vi "Signal-Generator.vi"() -> ()   [LabVIEW 2020]
uses:
  <vilib>/Analysis/1siggen.llb/Ramp Pattern by Samples.vi
  <vilib>/Analysis/2dsp.llb/Real FFT.vi
  <vilib>/Analysis/1siggen.llb/General Gauss-Mod Sine.vi
  <vilib>/Analysis/1siggen.llb/General Gaussian Monopulse.vi
  <vilib>/Analysis/1siggen.llb/General Aperiodic Triangle.vi
  <vilib>/Analysis/1siggen.llb/General Periodic Sinc.vi
  <vilib>/Analysis/NI_AALBase.lvlib
  <vilib>/Analysis/NI_AALPro.lvlib
panel:
  out "FFT":dbl[](graph)
  in  "dt":dbl=0.1
  in  "Delay":i32=50
  in  "SigFrequency":dbl=1.0 format="%.2f"
  in  "Samples":i32=256
  in  "Duration":dbl=1.0 format="%0.2f"
  in  "dc offset":dbl format="%0.2f"
  in  "Phase":dbl format="%0.2f"
  in  "Amplitude":dbl=1.0 format="%.2f"
  in  "Tab":T1(tab)
  in  "Duty (%)":dbl=50.0 format="%0.2f"
  in  "Width":i32=20
  in  "Am/Dm":cluster{"Am":dbl, "Dm":dbl}[](array[cluster])=[{"Am"=5.0, "Dm"=1.0}, {"Am"=3.0, "Dm"=8.0}, {"Am"=1.0, "Dm"=15.0}]
  in  "Interpolation":i32(ring)=1 items=["nearest", "linear", "spline", "cubic Hermite"]
  in  "Pluse":T2(ring)
  in  "f2":dbl=0.1 format="%0.2f"
  in  "f1":dbl=0.01 format="%0.2f"
  in  "Type":u16(ring) items=["Monopulse", "Gaussian Modulated Sine "]
  out "Graph":dbl[](graph)
  out "Error":i32
  out "Phase out":dbl format="%.2f"
  # "Common Parameters"
  # "Hz"
  # "Signal Generator"
  # "Instruction:\n1) Select signal from tab;\n2) Set parameters of selected signals;\n3) Run VI and check out the wave and frequency of the signal;\n4) Repeat step 1-3 to see other signal."
  # "Move phase of Sine wave 90degrees"
  # "Start=0;\nEnd=A"
  # "Start=A;\nEnd=0"
  # "Add Multi-tones and Gauss white noise"
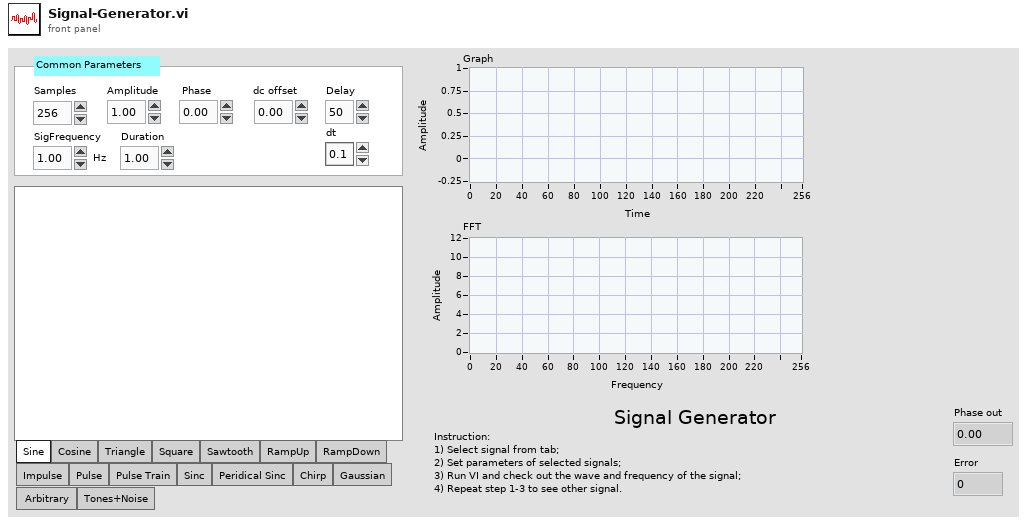
[diagram p1: front panel]
types:
  T1 = enum32{"Sine", "Cosine", "Triangle", "Square", "Sawtooth", "RampUp", "RampDown", "Impulse", "Pulse", "Pulse Train", "Sinc", "Peridical Sinc", "Chirp", "Gaussian", "Arbitrary ", "Tones+Noise"}
  T2 = enum16{"Gauss Mod-Sine", "Gauss Monopulse", "Triangle", "Sine", "Square", "Sinc"}
  T3 = cluster{"frequency":dbl, "amplitude":dbl, "phase":dbl}[]
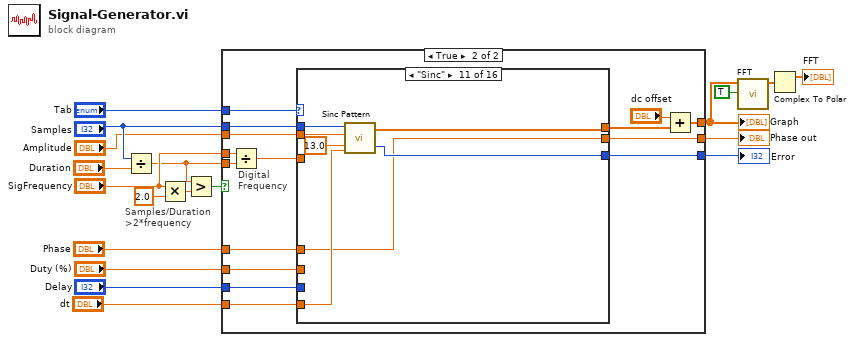
[diagram p0: block diagram]
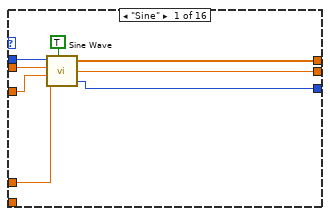
[diagram p3: hidden frame]
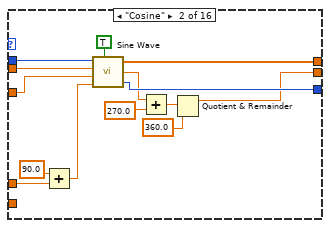
[diagram p4: hidden frame]
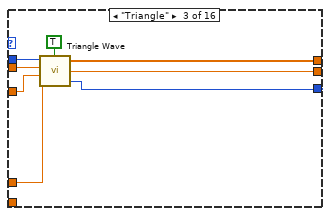
[diagram p5: hidden frame]
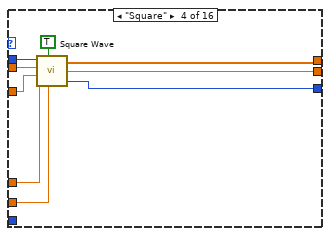
[diagram p6: hidden frame]
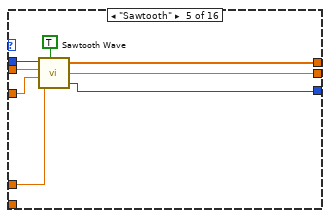
[diagram p7: hidden frame]
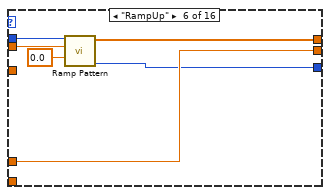
[diagram p8: hidden frame]
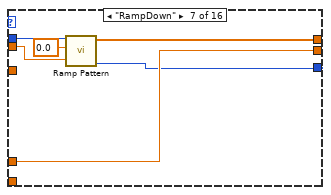
[diagram p9: hidden frame]
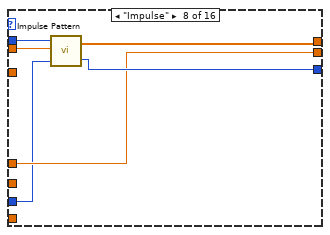
[diagram p10: hidden frame]
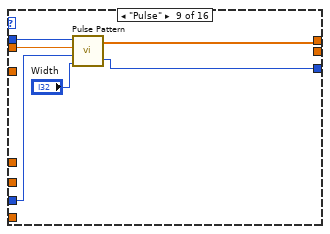
[diagram p11: hidden frame]
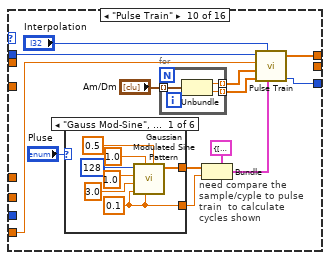
[diagram p12: hidden frame]
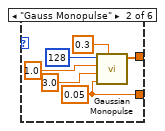
[diagram p13: hidden frame]
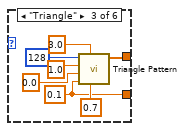
[diagram p14: hidden frame]
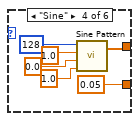
[diagram p15: hidden frame]
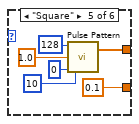
[diagram p16: hidden frame]
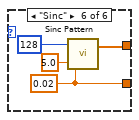
[diagram p17: hidden frame]
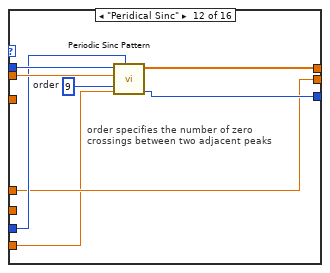
[diagram p18: hidden frame]
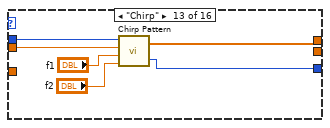
[diagram p19: hidden frame]
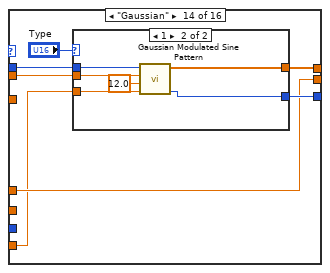
[diagram p20: hidden frame]
diagram:
  # "Samples/Duration \n>2*frequency"
  n1 = Divide(x="Samples", y="Duration") -> (x/y=w8:dbl)
  n2 = Multiply(x="SigFrequency", y=2.0) -> (x*y=w7:dbl)
  n3 = Greater?(x=w8, y=w7) -> (0:w11:bool)
  n4 = case shown="True" w11 {
    tunnel: w8 -> [_ w37]
    tunnel: "Samples" -> [_ w36]
    tunnel: "SigFrequency" -> [_ w26]
    tunnel: [-20061 ("error") w32] -> w19
    tunnel: [dbl[] [] ("Signal") w31] -> w4
    tunnel: "Tab" -> [_ w30]
    tunnel: "Amplitude" -> [_ w29]
    tunnel: "Phase" -> [w20 w28]
    tunnel: "Duty (%)" -> [_ w27]
    tunnel: [w20 w25] -> w12
    tunnel: "Delay" -> [_ w24]
    tunnel: "dt" -> [_ w23]
    frame False {
      # "Error: Nyquist Criterion violated\nsamples/duration must be > 2*frequency\nYou must adjust samples, duration, or frequency by:\n     increasing #samples\n     decreasing duration\n     decreasing frequency"
    }
    frame True {
      # "Digital \nFrequency"
      n5 = Divide(x=w26, y=w37) -> (x/y=w35:dbl)
      n6 = case shown="\"Sinc\"" w30 {
        tunnel: w29 -> [w45 w59 w67 w76 w78 w89 w93 w101 w108 _ w166 w175 w181 w188 w209 _]
        tunnel: w28 -> [w44 w46 w66 w75 w84 w86 w92 w98 _ _ w162 w169 _ w184 w206 _]
        tunnel: [w43 w55 w62 w69 w79 w87 w95 w99 w103 w119 w165 w170 w178 w185 w203 w212] -> w33
        tunnel: w36 -> [w42 w58 w65 w73 w83 w90 w96 w102 w107 w121 w167 w174 w180 w187 w208 w213]
        tunnel: w35 -> [w38 w48 w60 w74 w81 _ _ _ _ _ _ _ _ _ w207 _]
        tunnel: [w41 w50 w64 w72 w82 w86 w92 w98 _ _ w162 w169 _ w184 w204 _] -> w25
        tunnel: w27 -> [_ _ _ w71 _ _ _ _ _ _ _ _ _ _ _ _]
        tunnel: [w40 w54 w61 w68 w77 w85 w91 w100 w104 w120 w164 w171 w179 w186 w205 _] -> w32
        tunnel: w24 -> [_ _ _ _ _ _ _ w97 w106 _ _ w173 _ _ _ _]
        tunnel: w23 -> [_ _ _ _ _ _ _ _ _ w109 w163 w168 _ w183 _ _]
        frame "Sine" {
          n7 = call <vilib>:"Sine Wave.vi"("samples"=w42, "amplitude"=w45, "frequency"=w38, "phase in"=w44, "reset phase"=TRUE) -> ("sine wave"=w43:dbl[], "phase out"=w41:dbl, "error"=w40:i32)
        }
        frame "Cosine" {
          n8 = Add(x=90.0 ("y"), y=w46) -> (x+y=w56:dbl)
          n9 = call <vilib>:"Sine Wave.vi"("samples"=w58, "amplitude"=w59, "frequency"=w48, "phase in"=w56, "reset phase"=TRUE) -> ("sine wave"=w55:dbl[], "phase out"=w52:dbl, "error"=w54:i32)
          n10 = Add(x=w52, y=270.0) -> (x+y=w49:dbl)
          n11 = Quotient & Remainder(x=w49, y=360.0) -> (x-y*floor(x/y)=w50:dbl)  [unwired: 1 out]
        }
        frame "Triangle" {
          n12 = call <vilib>:"Triangle Wave.vi"("samples"=w65, "amplitude"=w67, "frequency"=w60, "phase in"=w66, "reset phase"=TRUE) -> ("triangle wave"=w62:dbl[], "phase out"=w64:dbl, "error"=w61:i32)
        }
        frame "Square" {
          n13 = call <vilib>:"Square Wave.vi"("samples"=w73, "reset phase"=TRUE, "amplitude"=w76, "frequency"=w74, "duty cycle (%)"=w71, "phase in"=w75) -> ("square wave"=w69:dbl[], "phase out"=w72:dbl, "error"=w68:i32)
        }
        frame "Sawtooth" {
          n14 = call <vilib>:"Sawtooth Wave.vi"("samples"=w83, "amplitude"=w78, "frequency"=w81, "phase in"=w84, "reset phase"=TRUE) -> ("sawtooth wave"=w79:dbl[], "phase out"=w82:dbl, "error"=w77:i32)
        }
        frame "RampUp" {
          n15 = call-poly <vilib>:"Ramp Pattern.vi"("start"=0.0, "end"=w89, "samples"=w90) -> ("error"=w85:i32, "Ramp Pattern"=w87:dbl[])  [unwired: 7 in]
        }
        frame "RampDown" {
          n16 = call-poly <vilib>:"Ramp Pattern.vi"("start"=w93, "end"=0.0 ("start"), "samples"=w96) -> ("error"=w91:i32, "Ramp Pattern"=w95:dbl[])  [unwired: 7 in]
        }
        frame "Impulse" {
          n17 = call <vilib>:"Impulse Pattern.vi"("delay"=w97, "amplitude"=w101, "samples"=w102) -> ("error"=w100:i32, "Impulse Pattern"=w99:dbl[])
        }
        frame "Pulse" {
          n18 = call <vilib>:"Pulse Pattern.vi"("width"="Width", "delay"=w106, "amplitude"=w108, "samples"=w107) -> ("error"=w104:i32, "Pulse Pattern"=w103:dbl[])
        }
        frame "Pulse Train" {
          # "need compare the sample/cyple to pulse train  to calculate cycles shown"
          n19 = case shown="\"Gauss Mod-Sine\", Default" "Pluse" {
            tunnel: [w128 w134 w138 w143 w153 w156] -> w110
            tunnel: [w122 w129 w137 0.05 0.1 ("delta t") w155] -> w113
            frame "Gauss Mod-Sine", Default {
              w122 = 0.1
              n20 = call <vilib>:"Gaussian Modulated Sine Pattern.vi"("attenuation (dB)"=0.5 ("attenuation"), "normalized bandwidth"=w122, "center frequency (Hz)"=1.0 ("center frequency"), "delta t (s)"=w122, "delay (s)"=3.0 ("delay"), "amplitude"=1.0, "samples"=128) -> ("Gauss-Mod Sine Pattern"=w128:dbl[])  [unwired: 3 in, 1 out]
            }
            frame "Gauss Monopulse" {
              w129 = 0.05 ("delta t")
              n21 = call <vilib>:"Gaussian Monopulse.vi"("center frequency (Hz)"=0.3 ("center frequency"), "delta t (s)"=w129, "delay (s)"=3.0 ("delay"), "amplitude"=1.0, "samples"=128) -> ("Gaussian Monopulse"=w134:dbl[])  [unwired: 5 in, 1 out]
            }
            frame "Triangle" {
              w137 = 0.1 ("delta t")
              n22 = call <vilib>:"Triangle Pattern.vi"("asymmetry"=0.7, "width (s)"=3.0 ("width"), "delta t (s)"=w137, "delay (s)"=0.0 ("delay"), "amplitude"=1.0, "samples"=128) -> ("Triangle Pattern"=w138:dbl[])  [unwired: 4 in, 1 out]
            }
            frame "Sine" {
              n23 = call <vilib>:"Sine Pattern.vi"("cycles"=1.0, "phase(degrees)"=0.0, "amplitude"=1.0, "samples"=128 ("samples 2")) -> ("Sinusoidal Pattern"=w143:dbl[])  [unwired: 1 out]
            }
            frame "Square" {
              n24 = call <vilib>:"Pulse Pattern.vi"("width"=10, "delay"=0, "amplitude"=1.0, "samples"=128) -> ("Pulse Pattern"=w153:dbl[])  [unwired: 1 out]
            }
            frame "Sinc" {
              w155 = 0.02 ("delta t")
              n25 = call <vilib>:"Sinc Pattern.vi"("delta t"=w155, "delay"=5.0, "samples"=128) -> ("Sinc Pattern"=w156:dbl[])  [unwired: 1 in, 1 out]
            }
          }
          n26 = for {
            tunnel: "Am/Dm" -> [w160] mode=indexing
            tunnel: [w159] -> w116 mode=indexing
            tunnel: [w158] -> w115 mode=indexing
            n27 = Unbundle(w160) -> ("Am"=w159:dbl, "Dm"=w158:dbl)
          }
          n28 = Bundle(cluster=cluster{"Sinusoidal Pattern":dbl[], dbl} {"Sinusoidal Pattern"=[], 0.0} ("output cluster"), "Sinusoidal Pattern"=w110, w113) -> (w112:cluster{"Sinusoidal Pattern":dbl[], dbl})
          n29 = call <vilib>:"Pulse Train.vi"("prototype spec"=w112, "interpolation method"="Interpolation", "Delay (s)"=w115, "Amplitude"=w116, "delta t of pulse train (s)"=w109, "samples"=w121) -> ("error"=w120:i32, "Pulse Train"=w119:dbl[])  [unwired: 4 in]
        }
        frame "Sinc" {
          n30 = call <vilib>:"Sinc Pattern.vi"("delta t"=w163, "delay"=13.0, "amplitude"=w166, "samples"=w167) -> ("error"=w164:i32, "Sinc Pattern"=w165:dbl[])
        }
        frame "Peridical Sinc" {
          w172 = 9  # order
          # "order specifies the number of zero \ncrossings between two adjacent peaks"
          n31 = call <vilib>:"Periodic Sinc Pattern.vi"("delay (s)"=w173, "delta t (s)"=w168, "order"=w172, "amplitude"=w175, "samples"=w174) -> ("error"=w171:i32, "Periodic Sinc Pattern"=w170:dbl[])  [unwired: 5 in]
        }
        frame "Chirp" {
          n32 = call <vilib>:"Chirp Pattern.vi"("f2"="f2", "f1"="f1", "amplitude"=w181, "samples"=w180) -> ("error"=w179:i32, "Chirp Pattern"=w178:dbl[])
        }
        frame "Gaussian" {
          n33 = case shown="1" "Type" {
            tunnel: w188 -> [w194 w198]
            tunnel: w187 -> [w193 w199]
            tunnel: [w192 w197] -> w186
            tunnel: [w191 w196] -> w185
            tunnel: w183 -> [w190 w200]
            frame 0, Default {
              n34 = call <vilib>:"Gaussian Monopulse.vi"("delta t (s)"=w190, "delay (s)"=12.0, "amplitude"=w194, "samples"=w193) -> ("error"=w192:i32, "Gaussian Monopulse"=w191:dbl[])  [unwired: 6 in]
            }
            frame 1 {
              n35 = call <vilib>:"Gaussian Modulated Sine Pattern.vi"("delta t (s)"=w200, "delay (s)"=12.0, "amplitude"=w198, "samples"=w199) -> ("error"=w197:i32, "Gauss-Mod Sine Pattern"=w196:dbl[])  [unwired: 6 in]
            }
          }
        }
        frame "Arbitrary " {
          w201 = 1 items=["none", "linear"]  # interpolation
          w202 = dbl[] [0.0, 1.0, 4.0, 1.0, 8.0, 6.0, 2.0, 1.0]  # Wave Table
          n36 = call <vilib>:"Arbitrary Wave.vi"("interpolation"=w201, "Wave Table"=w202, "phase in"=w206, "frequency"=w207, "amplitude"=w209, "samples"=w208) -> ("error"=w205:i32, "phase out"=w204:dbl, "arbitrary wave"=w203:dbl[])  [unwired: 1 in]
        }
        frame "Tones+Noise" {
          n37 = call <vilib>:"Tones and Noise.vi"("noise (rms)"=0.1, "tones"=T3 [{"frequency"=10.0, "amplitude"=5.0, "phase"=0.0}, {"frequency"=20.0, "amplitude"=0.1, "phase"=0.0}, {"frequency"=40.0, "amplitude"=1.0, "phase"=0.0}, {"frequency"=600.0, "amplitude"=2.0, "phase"=0.0}], "samples"=w213) -> ("tones and noise"=w212:dbl[])  [unwired: 7 in, 1 out]
        }
      }
      n38 = Add(x="dc offset", y=w33) -> (x+y=w31:dbl[])
    }
  }
  "Error" <- w19
  "Graph" <- w4
  "Phase out" <- w12
  n39 = call-poly <vilib>:"FFT.vi"("shift?"=TRUE, "X"=w4) -> ("FFT {X}"=w3:cdb[])  [unwired: 8 in, 1 out]
  n40 = Complex To Polar(r * e^(i*theta)=w3) -> (r=→"FFT":dbl[])  [unwired: 1 out]
